vi "ReleaseQueue.vi"(7 "Force Destroy? (F)":bool, 8 "error in (no error)":errorcluster, 11 "MessageQueue in":refnum<class "MessageQueue.lvclass">) -> (0 "error out":errorcluster, 2 "Remaining Messages":refnum<class "Message.lvclass">[](array[class]), 3 "Queue Name":string)   [LabVIEW 2009, in "LapDog.Messaging.v2.lvlib" / "MessageQueue.lvclass"]
doc: "Releases the MessageQueue and returns the remaining messages as an array.\n\nThis method executes regardless of the error in state."
uses:
  MessageQueue.lvclass
  MessageObject/Message.lvclass
  MessageQueue.lvclass/MessageQueue.ctl
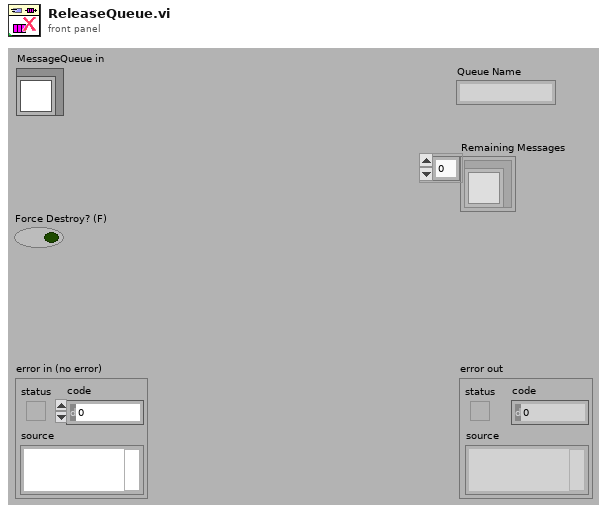
[diagram p1: front panel]
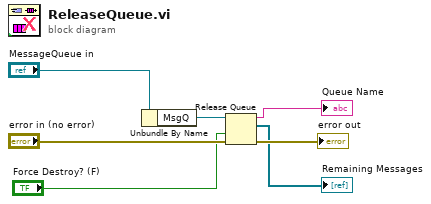
[diagram p0: block diagram]
diagram:
  n1 = Unbundle By Name("MessageQueue in") -> ("MsgQ"=w6:refnum<queue>)
  n2 = Release Queue(queue=w6, force destroy? (F)="Force Destroy? (F)", error in (no error)="error in (no error)") -> (queue name=→"Queue Name":string, remaining elements=→"Remaining Messages":refnum<class "Message.lvclass">[], error out=→"error out":errorcluster)
